vi "Host - 29x5 - 6592R Streaming.vi.LOCAL.vi"() -> ()   [LabVIEW 2016]
uses:
  <vilib>/userdefined/Silver/nirio_resource_slv.ctl
  TypeDefs/USRP Configuration.ctl
  29x5/SubVIs/Start Trigger.ctl
  TDMS Raw to Channels/Previewed Channel - Enum.ctl
  TypeDefs/States.ctl
  <instrlib>/niUsrpRio/Config/v1/Host/Public/niUsrpRio Session.ctl
  <instrlib>/_niInstr/Register Bus/v0/Host/Public/Register Bus Session.ctl
  <instrlib>/_niInstr/Register Bus/v0/Host/Private/Session Data.ctl
  <instrlib>/niUsrpRio/Config/v1/Host/Private/DB Queue Reference.ctl
  <instrlib>/niUsrpRio/Config/v1/Host/Private/Daughterboard Data.ctl
  <instrlib>/niUsrpRio/Config/v1/Host/Private/ATR state data.ctl
  <instrlib>/niUsrpRio/Config/v1/Host/Private/Antenna Configuration.ctl
  <instrlib>/niUsrpRio/Config/v1/Host/Private/CPLD Power Mode.ctl
  <instrlib>/niUsrpRio/Config/v1/Host/Public/EEPROM Header.ctl
  <instrlib>/niUsrpRio/Config/v1/Host/Public/EEPROM Device Data Header.ctl
  <instrlib>/niUsrpRio/Config/v1/Host/Public/EEPROM Characterization Header.ctl
  <instrlib>/niUsrpRio/Config/v1/Host/Public/Characterization Data.ctl
  <instrlib>/niUsrpRio/Config/v1/Host/Public/IQ Imbalance.ctl
  <vilib>/FPGAPlugInAG/Dynamic/niLvFpga_Close_Dynamic.vi
  <vilib>/rvi/interface/nirviCloseFPGA/nirviCloseFPGA.xnode
  <instrlib>/_niInstr/Register Bus/v0/Host/niInstr Register Bus v0 Host.lvlib
  <instrlib>/niUsrpRio/Config/v1/Host/niUsrpRio Config v1 Host.lvlib
panel:
  in  "Previewed Channel":T1
  in  "Exit":bool
  in  "Stop":bool
  in  "Run":bool
  out "Throughput (B/s)":dbl[](array[numeric]) format="%#.3p"
  out "Power Spectral Density (PSD)":cluster{"f0":dbl, "df":dbl, "magnitude":dbl[]}(graph)
  in  "File Path":path=path "D:/USRP Project TDMS Files"
  in  "USRP Configuration":T2={"USRP RIO Resources"=["USRP-2945"], "LO Sharing"=TRUE, "Carrier Frequency (Hz)"=2000000000.0, "Gain"=40.0, "Sample rate (Hz)"=100000000.0, "reference frequency source"="Internal", "start trigger"=enum."Software"} {"Sample rate (Hz)" format="%#_6p"; "Carrier Frequency (Hz)" format="%#_6p"}
  in  "Simulate Data":bool
  in  "6592R Resources":T3[](array[typedef])=["High_Speed_Module"]
  # "Hardware Settings"
  # "Recording Settings"
  # "Todos: \n- Make the UI fit into 1 screen!\n- General Hints for the user on how to \nrun the code\n- if \"stop\" button is pressed, \"quit\" ist grayed out"
  # "Channel Preview"
  # "TwinRx Aurora - 4 Channel Record Demo"
  # "Control Demo"
  # "Throughput (B/s)"
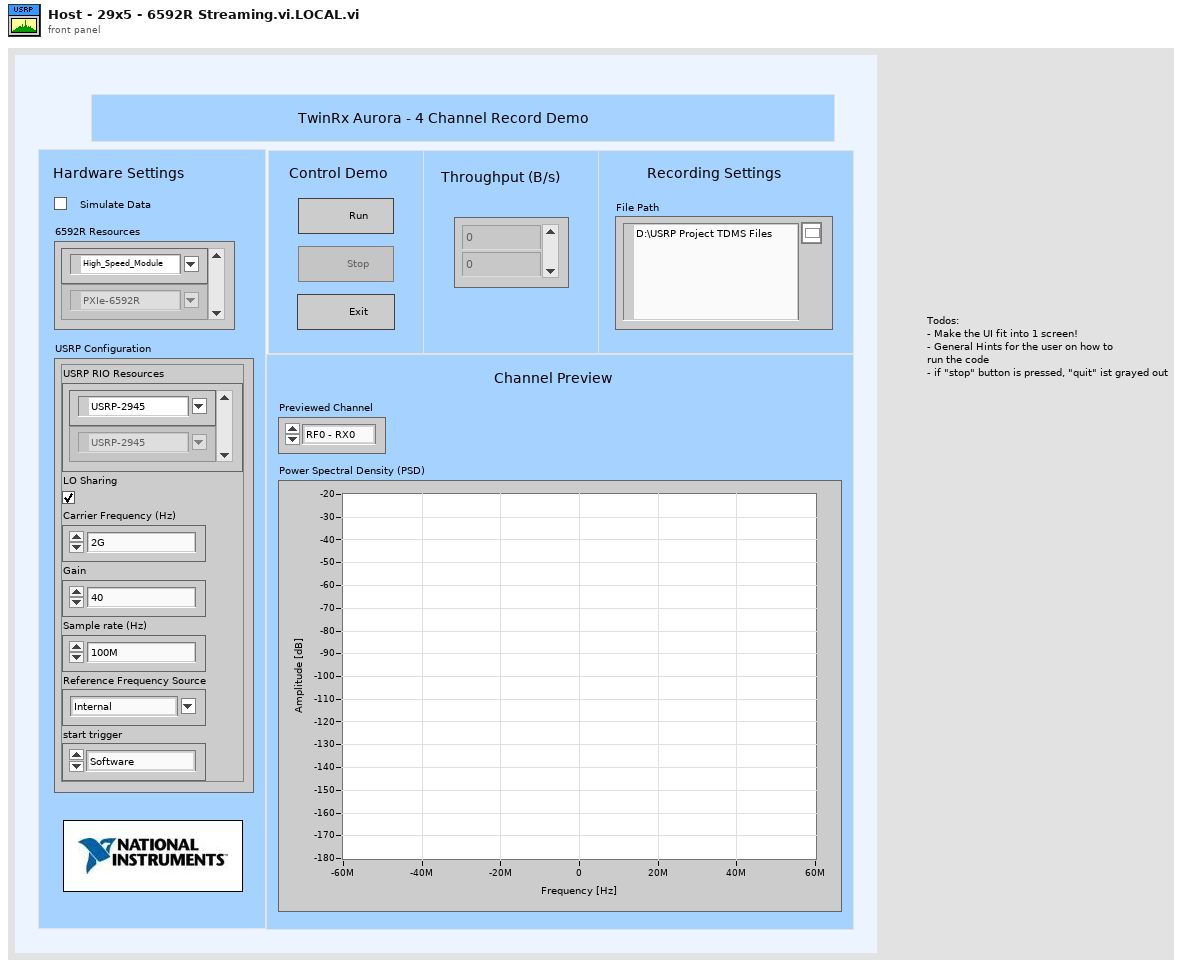
[diagram p1: front panel]
types:
  T1 = typedef "Previewed Channel - Enum.ctl" = enum16{"RF0 - RX0", "RF0 - RX1", "RF1 - RX0", "RF1 - RX1"}
  T2 = typedef "USRP Configuration.ctl" = cluster{"USRP RIO Resources":T3[], "LO Sharing":bool, "Carrier Frequency (Hz)":dbl, "Gain":dbl, "Sample rate (Hz)":dbl, "reference frequency source":string, "start trigger":T4}
  T3 = typedef "nirio_resource_slv.ctl" = tag
  T4 = typedef "Start Trigger.ctl" = enum8{"Software", "Digital Edge", "Rx Start Trigger", "Tx Start Trigger", "Immediate", "Future Time Event"}
  T5 = typedef "niUsrpRio Config v1 Host.lvlib/niUsrpRio Session.ctl" = cluster{"FPGA Interface":refnum<k20>, "RIO Interface Number":u32, "Data Clock Rate":u32, "FPGA Data Clock Rate":u32, "Global Settings Register Bus":T6, "Radio 0 Settings Register Bus":T6, "Radio 1 Settings Register Bus":T6, "Radio Settings Bus Semaphore":T7, "DB Queues":T8[], "Characterization Data Valid?":bool, "EEPROM Header":T9, "Device Data Header":T10, "EEPROM Characterization Header":T11, "Characterization Data":T12[], "FPGA Current Version":u32, "FPGA Oldest Compatible Version":u32, "Fixed Logic Current Version":u32, "Fixed Logic Oldest Compatible Version":u32, "FPGA Radio Settings Bus Current Version":u32, "FPGA Radio Settings Bus Oldest Compatible Version":u32, "FPGA Board Config Current Version":u32, "FPGA Board Config Oldest Compatible Version":u32, "Daughterboard Clock Rate":u32, "daughterboard configuration session handles":u64[]}
  T6 = typedef "niInstr Register Bus v0 Host.lvlib/Register Bus Session.ctl" = refnum<queue>
  T7 = typedef "Semaphore RefNum" = refnum<k1>
  T8 = typedef "niUsrpRio Config v1 Host.lvlib/DB Queue Reference.ctl" = refnum<queue>
  T9 = typedef "niUsrpRio Config v1 Host.lvlib/EEPROM Header.ctl" = cluster{"Checksum":u32, "Product Code":u16, "Hardware Current Version":u16, "Hardware Oldest Compatible Version":u16, "EEPROM Map Current Version":u16, "EEPROM Map Oldest Compatible Version":u16, "User Password":string, "Pointer to Factory Header":u32, "Pointer to User Header":u32, "Recommended Interval":u16, "Number of Reserved Bytes":i32, "Number of Daughterboards":u8, "Daughterboard IDs":u16[], "Daughterboard Serial Numbers":string[]}
  T10 = typedef "niUsrpRio Config v1 Host.lvlib/EEPROM Device Data Header.ctl" = cluster{"Checksum":u32, "Number of Channels":u8, "Number of Gain Settings":u16[], "Pointer to Characterization Data":u32[], "Number of Reserved Bytes":i32, "Number of Frequencies":u16[]}
  T11 = typedef "niUsrpRio Config v1 Host.lvlib/EEPROM Characterization Header.ctl" = cluster{"Checksum":u32, "Date":timestamp, "Temperature":sgl, "Misc. Info":string, "Pointer to Device Data Header":u32, "Number of Reserved Bytes":i32}
  T12 = typedef "niUsrpRio Config v1 Host.lvlib/Characterization Data.ctl" = cluster{"Gains[dB]":dbl[], "Frequencies [Hz]":dbl[], "IQ Imbalance Table":T13[], "Measured Gains[dB]":dbl[][]}
  T13 = typedef "niUsrpRio Config v1 Host.lvlib/IQ Imbalance.ctl" = cluster{"Gain Imbalance [linear]":dbl, "Phase Imbalance [radians]":dbl, "Offset":cdb}
  T14 = cluster{"HS-Serial Resource":T3[], "USRP Configuration":T2, "File Path":path, "Refnum out":refnum<k20>[], "2 USRPs?":bool[], "niUsrpRio Session":T5[], "TDMS Refnum":refnum<k34>, "Simulate Data?":bool}
  T15 = typedef "States.ctl" = enum16{"Choose Settings", "Exit", "Configure", "Run", "Close", "Shutdown", "transition to Run"}
  T16 = enum8{"Enabled", "Disabled", "Disabled and Grayed Out"}
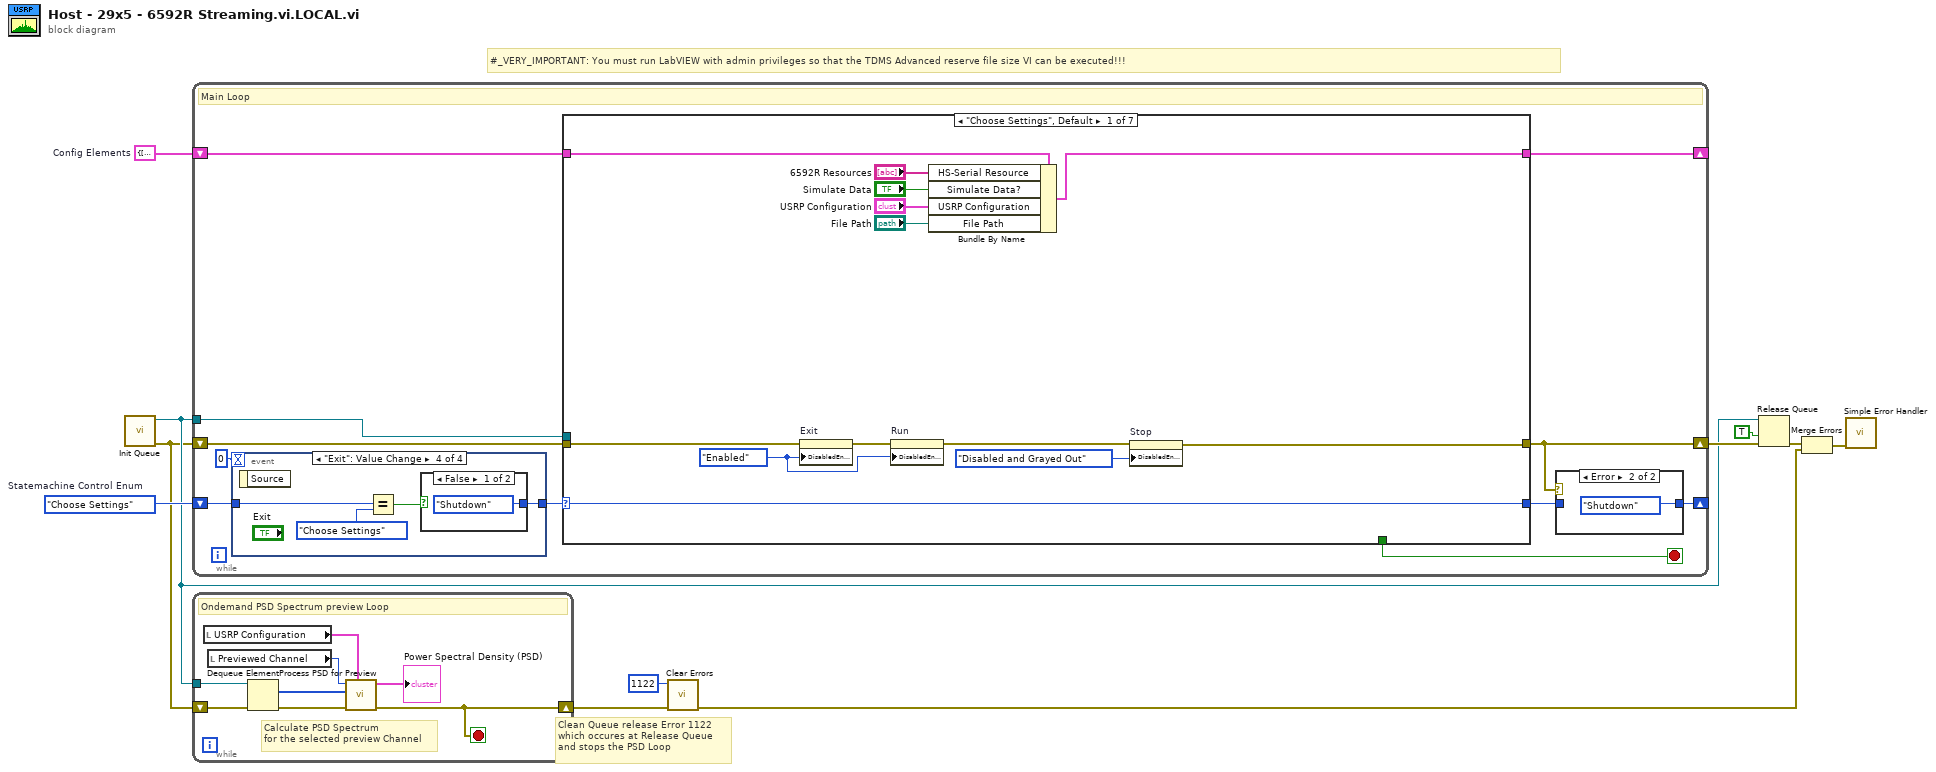
[diagram p0: block diagram]
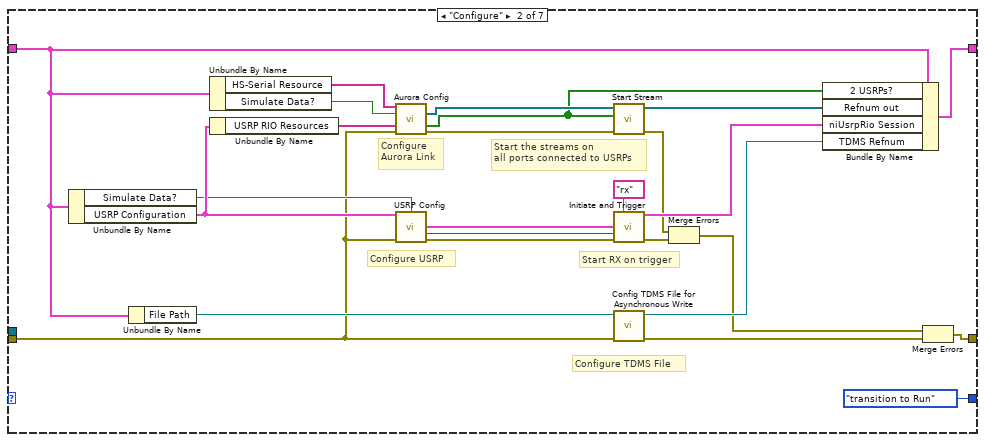
[diagram p3: hidden frame]
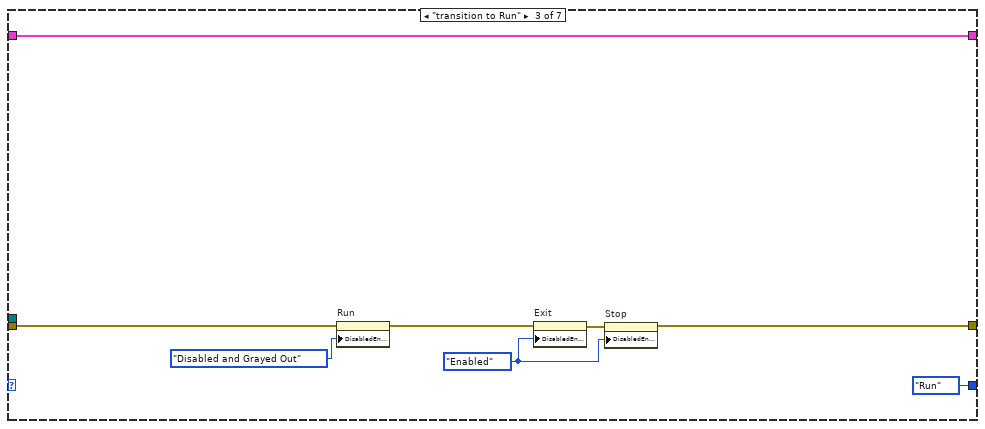
[diagram p4: hidden frame]
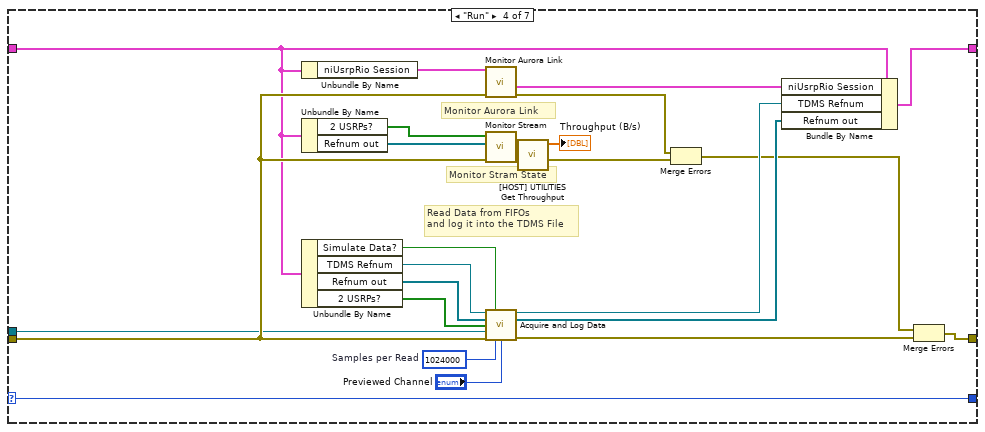
[diagram p5: hidden frame]
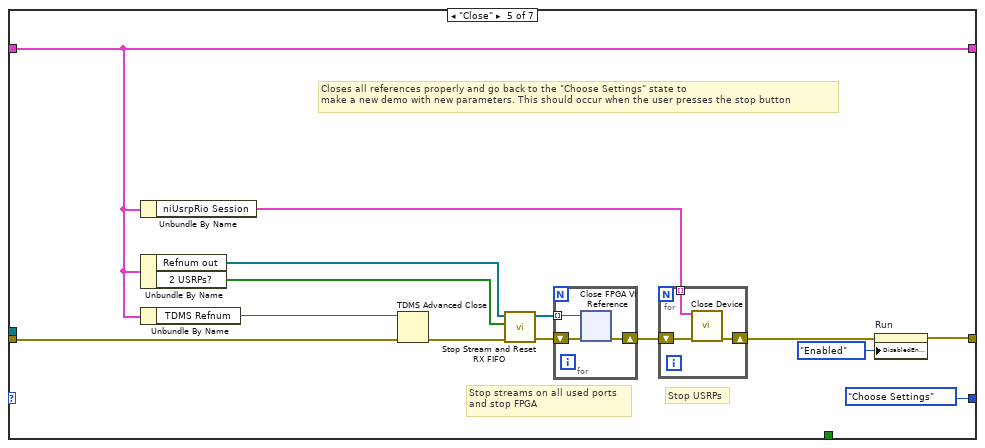
[diagram p6: hidden frame]
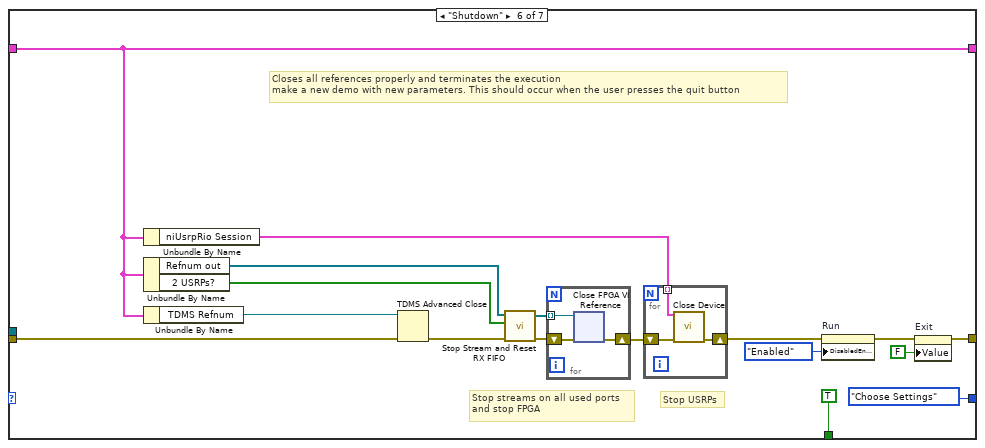
[diagram p7: hidden frame]
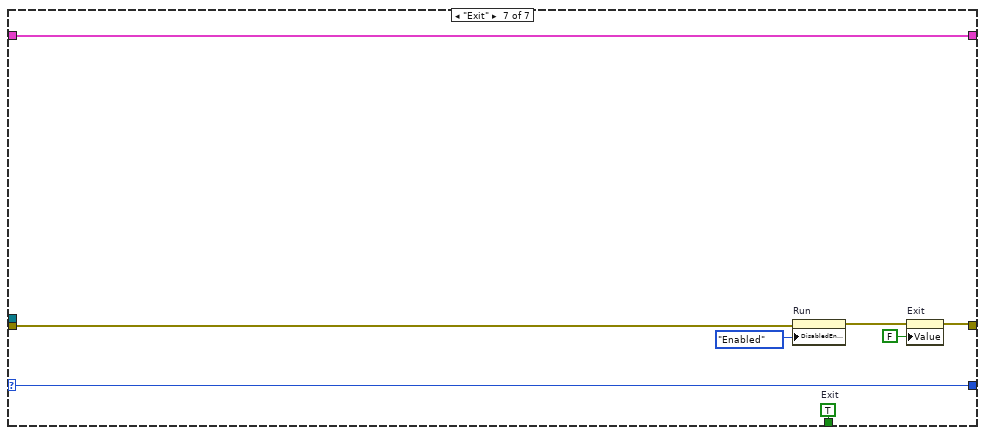
[diagram p8: hidden frame]
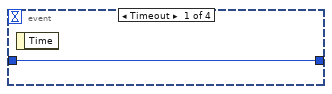
[diagram p9: hidden frame]
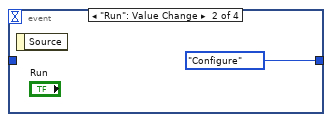
[diagram p10: hidden frame]
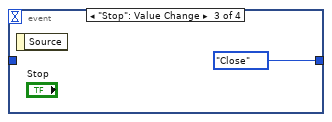
[diagram p11: hidden frame]
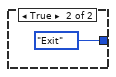
[diagram p12: hidden frame]
diagram:
  w10 = T14 {"HS-Serial Resource"=[], "USRP Configuration"={"USRP RIO Resources"=["USRP-2945"], "LO Sharing"=TRUE, "Carrier Frequency (Hz)"=2000000000.0, "Gain"=40.0, "Sample rate (Hz)"=100000000.0, "reference frequency source"="Internal", "start trigger"=enum."Software"}, "File Path"=path "", "Refnum out"=[], "2 USRPs?"=[], "niUsrpRio Session"=[], "TDMS Refnum"=refnum, "Simulate Data?"=FALSE}  # Config Elements
  w11 = States."Choose Settings"  # Statemachine Control Enum
  # "Clean Queue release Error 1122\nwhich occures at Release Queue \nand stops the PSD Loop"
  # "#_VERY_IMPORTANT: You must run LabVIEW with admin privileges so that the TDMS Advanced reserve file size VI can be executed!!!"
  n1 = call "Init Queue.vi"() -> ("error out"=w3:errorcluster, "Queue out"=w4:refnum<queue>)  [unwired: 10 in]
  n2 = while {
    shift-right: [w16] -> _
    shift-left: w11 -> [w22]
    shift-right: [w15] -> w9
    shift-left: w3 -> [w19]
    shift-right: [w13] -> _
    shift-left: w10 -> [w14]
    tunnel: w4 -> [w12]
    stop <- w18 stop-if-true
    # "Main Loop"
    n3 = event shown="[3] \"Exit\": Value Change" {
      selector: _ -> [_ _ _ _]
      dyn-events: _ -> [_ _ _ _]
      timeout: 0 -> [_ _ _ _]
      tunnel: [w147 States."Configure" States."Close" w151] -> w21
      tunnel: w22 -> [w147 _ _ w152]
      event Timeout {
        n4 = event-data() -> ()  [unwired: 1 in, 1 out]
      }
      event "Run": Value Change {
        n5 = event-data() -> ()  [unwired: 1 in, 1 out]
      }
      event "Stop": Value Change {
        n6 = event-data() -> ()  [unwired: 1 in, 1 out]
      }
      event "Exit": Value Change {
        n7 = event-data() -> ()  [unwired: 1 in, 1 out]
        n8 = Equal?(x=w152, y=States."Choose Settings") -> (x = y?=w150:bool)
        n9 = case shown="False" w150 {
          tunnel: [States."Shutdown" States."Exit"] -> w151
          frame False {
          }
          frame True {
          }
        }
      }
    }
    n10 = case shown="\"Choose Settings\", Default" w21 {
      selector: w21 -> [w26 _ _ w92 _ _ w139]
      tunnel: [w25 w45 w70 w81 w97 w118 w143] -> w15
      tunnel: [w26 States."transition to Run" States."Run" w92 States."Choose Settings" States."Choose Settings" w139] -> w17
      tunnel: w19 -> [w31 w43 w67 w95 w107 w130 w140]
      tunnel: [_ _ _ _ _ TRUE w145] -> w18
      tunnel: w14 -> [w37 w52 w69 w84 w99 w122 w146]
      tunnel: [w32 w49 w69 w80 w99 w122 w146] -> w13
      tunnel: w12 -> [_ _ _ w72 _ _ _]
      frame "Choose Settings", Default {
        w30 = T16."Enabled" ("Disabled")
        n11 = property on="Exit" class="Bool (strict)"(error in=w31, "DisabledEnum"=w30) -> (error out=w29:errorcluster)  [unwired: 1 in, 1 out]
        n12 = property on="Run" class="Bool"(error in=w29, "DisabledEnum"=w30) -> (error out=w28:errorcluster)  [unwired: 1 in, 1 out]
        n13 = Bundle By Name(cluster=w37, "HS-Serial Resource"="6592R Resources", "Simulate Data?"="Simulate Data", "USRP Configuration"="USRP Configuration", "File Path"="File Path") -> (w32:T14)
        n14 = property on="Stop" class="Bool"(error in=w28, "DisabledEnum"=T16."Disabled and Grayed Out" ("Disabled")) -> (error out=w25:errorcluster)  [unwired: 1 in, 1 out]
      }
      frame "Configure" {
        # "Start RX on trigger"
        # "Configure TDMS File"
        # "Start the streams on \nall ports connected to USRPs"
        # "Configure \nAurora Link"
        # "Configure USRP"
        n15 = Unbundle By Name(w52) -> ("Simulate Data?"=w54:bool, "USRP Configuration"=w57:T2)
        n16 = Unbundle By Name(w52) -> ("File Path"=w53:path)
        n17 = Unbundle By Name(w52) -> ("HS-Serial Resource"=w56:T3[], "Simulate Data?"=w55:bool)
        n18 = Unbundle By Name(w57) -> ("USRP RIO Resources"=w63:T3[])
        n19 = call "Aurora Config.vi"("6592R Resources"=w56, "Simulate and check Data"=w55, "USRP RIO Resources"=w63, "error in (no error)"=w43) -> ("Refnum out"=w48:refnum<k20>[], "2 USRPs?"=w38:bool[], "error out"=w47:errorcluster)  [unwired: 8 in, 1 out]
        n20 = call "USRP Config.vi"("USRP Configuration"=w57, "Simulate and check Data"=w54, "error in (no error)"=w43) -> ("Array"=w61:T5[], "start trigger out"=w60:T4, "Time Stamp"=w59:timestamp, "error out"=w46:errorcluster)  [unwired: 7 in, 2 out]
        n21 = call "Start Stream.vi"("error in (no error)"=w47, "2 USRPs?"=w38, "Refnum in"=w48) -> ("error out"=w41:errorcluster, "Refnum out"=w39:refnum<k20>[])  [unwired: 7 in]
        n22 = call "Initiate and Trigger.vi"("niUsrpRio Sessions"=w61, "scope"="rx", "start trigger"=w60, "start trigger time"=w59, "error in"=w46) -> ("niUsrpRio Sessions (out)"=w51:T5[], "error out"=w42:errorcluster)  [unwired: 9 in]
        n23 = call "Config TDMS File for Asynchronous Write.vi"("error in (no error)"=w43, "base path"=w53) -> ("error out"=w44:errorcluster, "Refnum out"=w50:refnum<k34>)  [unwired: 8 in]
        n24 = Merge Errors(w41, w42) -> (w40:errorcluster)
        n25 = Bundle By Name(cluster=w52, "2 USRPs?"=w38, "Refnum out"=w39, "niUsrpRio Session"=w51, "TDMS Refnum"=w50) -> (w49:T14)
        n26 = Merge Errors(w40, w44) -> (w45:errorcluster)
      }
      frame "transition to Run" {
        w68 = T16."Enabled" ("Disabled")
        n27 = property on="Run" class="Bool"(error in=w67, "DisabledEnum"=T16."Disabled and Grayed Out" ("Disabled")) -> (error out=w66:errorcluster)  [unwired: 1 in, 1 out]
        n28 = property on="Exit" class="Bool (strict)"(error in=w66, "DisabledEnum"=w68) -> (error out=w71:errorcluster)  [unwired: 1 in, 1 out]
        n29 = property on="Stop" class="Bool"(error in=w71, "DisabledEnum"=w68) -> (error out=w70:errorcluster)  [unwired: 1 in, 1 out]
      }
      frame "Run" {
        w73 = u32 1024000  # Samples per Read
        # "Read Data from FIFOs \nand log it into the TDMS File"
        # "Monitor Stram State"
        # "Monitor Aurora Link"
        n30 = Unbundle By Name(w84) -> ("niUsrpRio Session"=w91:T5[])
        n31 = Unbundle By Name(w84) -> ("2 USRPs?"=w90:bool[], "Refnum out"=w89:refnum<k20>[])
        n32 = Unbundle By Name(w84) -> ("Simulate Data?"=w88:bool, "TDMS Refnum"=w87:refnum<k34>, "Refnum out"=w86:refnum<k20>[], "2 USRPs?"=w85:bool[])
        n33 = call "Monitor Aurora Link.vi"("error in (no error)"=w95, "niUsrpRio Sessions (In)"=w91) -> ("error out"=w76:errorcluster, "niUsrpRio Sessions (Out)"=w83:T5[])  [unwired: 6 in, 2 out]
        n34 = call "Monitor Stream.vi"("error in (no error)"=w95, "Refnum in"=w89, "2 USRPs?"=w90) -> ("error out"=w77:errorcluster, "Samples Transferred"=w93:u64[])  [unwired: 6 in, 1 out]
        n35 = call "Acquire and Log Data.vi"("TDMS Refnum in"=w87, "Simulate Data"=w88, "Refnum in"=w86, "2 USRPs?"=w85, "Data Queue in"=w72, "error in (no error)"=w95, "Samples per Read"=w73, "Previewed Channel"="Previewed Channel") -> ("TDMS Refnum out"=w79:refnum<k34>, "Refnum out"=w82:refnum<k20>[], "error out"=w74:errorcluster)  [unwired: 5 in]
        n36 = call "[HOST] UTILITIES Get Throughput.vi"("Samples"=w93) -> ("Throughput"=→"Throughput (B/s)":dbl[])  [unwired: 10 in]
        n37 = Merge Errors(w76, w77) -> (w75:errorcluster)
        n38 = Bundle By Name(cluster=w84, "niUsrpRio Session"=w83, "TDMS Refnum"=w79, "Refnum out"=w82) -> (w80:T14)
        n39 = Merge Errors(w75, w74) -> (w81:errorcluster)
      }
      frame "Close" {
        # "Closes all references properly and go back to the \"Choose Settings\" state to \nmake a new demo with new parameters. This should occur when the user presses the stop button"
        # "Stop streams on all used ports \nand stop FPGA"
        # "Stop USRPs"
        n40 = Unbundle By Name(w99) -> ("niUsrpRio Session"=w100:T5[])
        n41 = Unbundle By Name(w99) -> ("Refnum out"=w102:refnum<k20>[], "2 USRPs?"=w101:bool[])
        n42 = Unbundle By Name(w99) -> ("TDMS Refnum"=w103:refnum<k34>)
        n43 = TDMS Advanced Close(8:w107, 11:w103) -> (0:w106:errorcluster)  [unwired: 2 in, 1 out]
        n44 = call "Stop Stream and Reset RX FIFO.vi"("error in (no error)"=w106, "2 USRPs?"=w101, "Refnum in"=w102) -> ("error out"=w108:errorcluster, "Refnum out"=w109:refnum<k20>[])  [unwired: 7 in]
        n45 = for {
          tunnel: w109 -> [w114] mode=indexing
          shift-right: [w115] -> w105
          shift-left: w108 -> [w113]
          n46 = xnode "Close FPGA VI Reference"("FPGA VI Reference In"=w114, "error in"=w113) -> ("error out"=w115:errorcluster)
        }
        n47 = for {
          shift-right: [w111] -> w96
          shift-left: w105 -> [w112]
          tunnel: w100 -> [w110] mode=indexing
          n48 = call "Close Device.vi"("niUsrpRio Session"=w110, "error in"=w112) -> ("error out"=w111:errorcluster)  [unwired: 13 in]
        }
        n49 = property on="Run" class="Bool"(error in=w96, "DisabledEnum"=T16."Enabled" ("Disabled")) -> (error out=w97:errorcluster)  [unwired: 1 in, 1 out]
      }
      frame "Shutdown" {
        # "Stop streams on all used ports \nand stop FPGA"
        # "Closes all references properly and terminates the execution\nmake a new demo with new parameters. This should occur when the user presses the quit button"
        # "Stop USRPs"
        n50 = Unbundle By Name(w122) -> ("niUsrpRio Session"=w123:T5[])
        n51 = Unbundle By Name(w122) -> ("Refnum out"=w125:refnum<k20>[], "2 USRPs?"=w124:bool[])
        n52 = Unbundle By Name(w122) -> ("TDMS Refnum"=w126:refnum<k34>)
        n53 = TDMS Advanced Close(8:w130, 11:w126) -> (0:w129:errorcluster)  [unwired: 2 in, 1 out]
        n54 = call "Stop Stream and Reset RX FIFO.vi"("error in (no error)"=w129, "2 USRPs?"=w124, "Refnum in"=w125) -> ("error out"=w131:errorcluster, "Refnum out"=w132:refnum<k20>[])  [unwired: 7 in]
        n55 = for {
          tunnel: w132 -> [w137] mode=indexing
          shift-right: [w138] -> w128
          shift-left: w131 -> [w136]
          n56 = xnode "Close FPGA VI Reference"("FPGA VI Reference In"=w137, "error in"=w136) -> ("error out"=w138:errorcluster)
        }
        n57 = for {
          shift-right: [w134] -> w116
          shift-left: w128 -> [w135]
          tunnel: w123 -> [w133] mode=indexing
          n58 = call "Close Device.vi"("niUsrpRio Session"=w133, "error in"=w135) -> ("error out"=w134:errorcluster)  [unwired: 13 in]
        }
        n59 = property on="Run" class="Bool"(error in=w116, "DisabledEnum"=T16."Enabled" ("Disabled")) -> (error out=w117:errorcluster)  [unwired: 1 in, 1 out]
        n60 = property on="Exit" class="Bool (strict)"(error in=w117, "Value"=FALSE ("Exit")) -> (error out=w118:errorcluster)  [unwired: 1 in, 1 out]
      }
      frame "Exit" {
        w145 = TRUE  # Exit
        n61 = property on="Run" class="Bool"(error in=w140, "DisabledEnum"=T16."Enabled" ("Disabled")) -> (error out=w141:errorcluster)  [unwired: 1 in, 1 out]
        n62 = property on="Exit" class="Bool (strict)"(error in=w141, "Value"=FALSE ("Exit")) -> (error out=w143:errorcluster)  [unwired: 1 in, 1 out]
      }
    }
    n63 = case shown="Error" w15 {
      tunnel: [w23 States."Shutdown"] -> w16
      tunnel: w17 -> [w23 _]
      frame No Error {
      }
      frame Error {
      }
    }
  }
  n64 = while {
    shift-right: [w156] -> w5
    shift-left: w3 -> [w163]
    tunnel: w4 -> [w161]
    stop <- w156 stop-if-true
    # "Calculate PSD Spectrum\nfor the selected preview Channel"
    # "Ondemand PSD Spectrum preview Loop"
    n65 = local read "USRP Configuration"() -> (w157:T2)
    n66 = local read "Previewed Channel"() -> (w159:T1)
    n67 = Dequeue Element(queue=w161, error in (no error)=w163) -> (element=w158:u64[], error out=w162:errorcluster)  [unwired: 1 in, 2 out]
    n68 = call "Process PSD for Preview.vi"("USRP Configuration"=w157, "error in (no error)"=w162, "Data Array"=w158, "Previewed Channel"=w159) -> ("error out"=w156:errorcluster, "Power Spectrum / PSD"=→"Power Spectral Density (PSD)":cluster{"f0":dbl, "df":dbl, "magnitude":dbl[]})  [unwired: 6 in]
  }
  n69 = call <vilib>:"Clear Errors.vi"("error in (no error)"=w5, "specific error code to clear (0: all)"=1122) -> ("error out"=w2:errorcluster)  [unwired: 4 in, 1 out]
  n70 = Release Queue(queue=w4, force destroy? (F)=TRUE, error in (no error)=w9) -> (error out=w7:errorcluster)  [unwired: 2 out]
  n71 = Merge Errors(w7, w2) -> (w6:errorcluster)
  n72 = call <vilib>:"Simple Error Handler.vi"("error in (no error)"=w6) -> ()  [unwired: 4 in, 5 out]
